vi "Read Typedef Path.vi"(8 "error in (no error)":errorcluster, 11 "Simple Struct Writer in":refnum<class "Simple Struct Writer.lvclass">) -> (0 "error out":errorcluster, 2 "Typedef Path":path, 3 "Simple Struct Writer out":refnum<class "Simple Struct Writer.lvclass">)   [LabVIEW 2013, in "Simple Struct Writer.lvclass"]
uses:
  Simple Struct Writer.lvclass
  Simple Struct Writer.lvclass/Simple Struct Writer.ctl
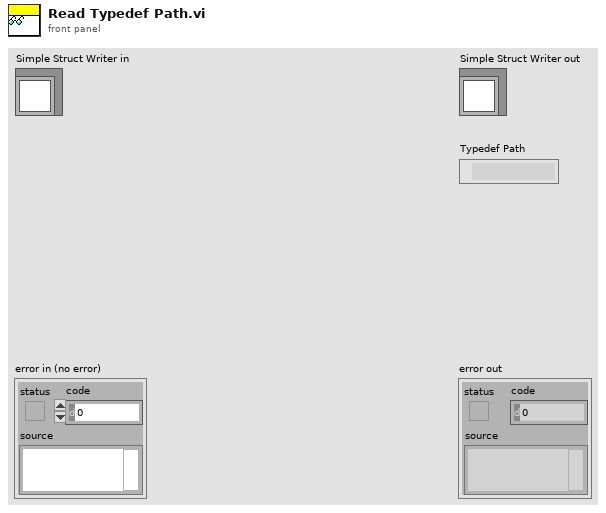
[diagram p1: front panel]
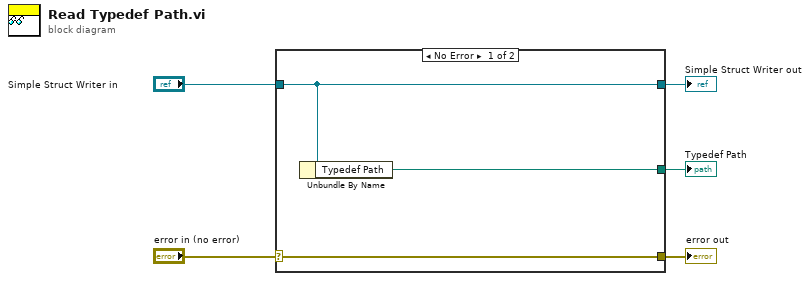
[diagram p0: block diagram]
diagram:
  n1 = case shown="No Error" "error in (no error)" {
    selector: "error in (no error)" -> [w8 w9]
    tunnel: [w8 w9] -> w4
    tunnel: [w7 w10] -> w2
    tunnel: "Simple Struct Writer in" -> [w7 w10]
    tunnel: [w6 _] -> w1
    frame No Error {
      n2 = Unbundle By Name(w7) -> ("Typedef Path"=w6:path)
    }
    frame Error {
    }
  }
  "error out" <- w4
  "Simple Struct Writer out" <- w2
  "Typedef Path" <- w1
